vi "get cipher core.vi"(8 "error in":errorcluster, 11 "cipher name":string) -> (0 "error out":errorcluster, 2 "sizes":T1, 3 "cipher":u64)   [LabVIEW 2016, in "lvlibcrypto cipher.lvclass"]
uses:
  lvlibcrypto cipher.lvclass
  lv tls dll.lvlib
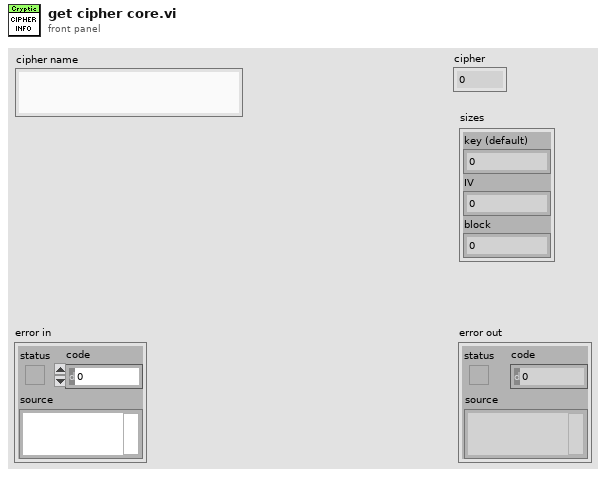
[diagram p1: front panel]
types:
  T1 = cluster{"key (default)":i32, "IV":i32, "block":i32}
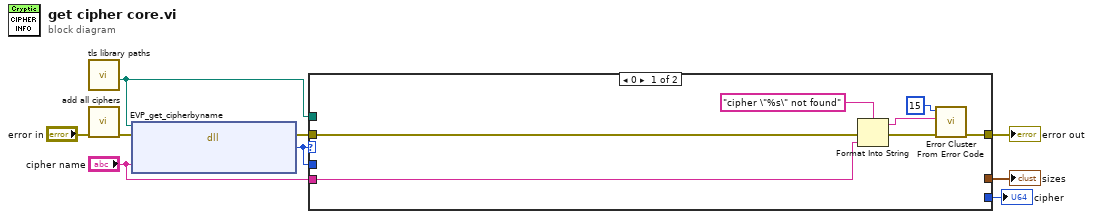
[diagram p0: block diagram]
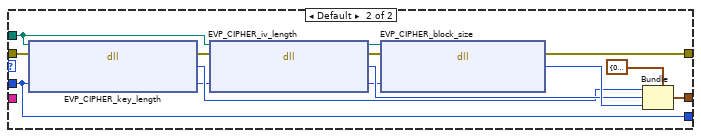
[diagram p2: hidden frame]
diagram:
  n1 = call "tls library paths.vi"() -> ("libcrypto"=w3:path)  [unwired: 8 in, 3 out]
  n2 = call "add all ciphers.vi"("error in"="error in") -> ("error out"=w4:errorcluster)  [unwired: 10 in]
  n3 = dll-call lib="C:/Users/IEUser/Desktop/tlssimple/libcrypto-41.dll" fn="EVP_get_cipherbyname"(path in=w3, error in=w4, "cipher name"="cipher name") -> (error out=w9:errorcluster, "cipher"=w6:u64)  [unwired: 2 in, 1 out]
  n4 = case shown="0" w6 {
    tunnel: w9 -> [w16 w29]
    tunnel: w3 -> [_ w26]
    tunnel: [w15 w30] -> w8
    tunnel: "cipher name" -> [w11 _]
    tunnel: w6 -> [_ w17]
    tunnel: [_ w20] -> w2
    tunnel: [_ w17] -> w1
    frame 0 {
      n5 = Format Into String(format string="cipher \"%s\" not found", error in=w16, w11) -> (resulting string=w12:string, error out=w13:errorcluster)  [unwired: 1 in]
      n6 = call <vilib>:"Error Cluster From Error Code.vi"("error in (no error)"=w13, "error message (\"\")"=w12, "error code (0)"=15) -> ("error out"=w15:errorcluster)  [unwired: 6 in]
    }
    frame Default {
      n7 = dll-call lib="C:/Users/IEUser/Desktop/tlssimple/libcrypto-41.dll" fn="EVP_CIPHER_key_length"(path in=w26, error in=w29, "cipher"=w17) -> (error out=w27:errorcluster, "size"=w21:i32, "cipher"=w19:u64)  [unwired: 1 in, 1 out]
      n8 = dll-call lib="C:/Users/IEUser/Desktop/tlssimple/libcrypto-41.dll" fn="EVP_CIPHER_iv_length"(path in=w26, error in=w27, "cipher"=w19) -> (path out=w25:path, error out=w28:errorcluster, "size"=w22:i32, "cipher"=w18:u64)  [unwired: 1 in]
      n9 = dll-call lib="C:/Users/IEUser/Desktop/tlssimple/libcrypto-41.dll" fn="EVP_CIPHER_block_size"(path in=w25, error in=w28, "cipher"=w18) -> (error out=w30:errorcluster, "size"=w23:i32)  [unwired: 2 in, 1 out]
      n10 = Bundle(cluster=T1 {"key (default)"=0, "IV"=0, "block"=0} ("sizes"), "key (default)"=w21, "IV"=w22, "block"=w23) -> (w20:T1)
    }
  }
  "error out" <- w8
  "sizes" <- w2
  "cipher" <- w1
